vi "UpdateVacPLC.vi"(0 "index of element":i32, 2 "DIMControlMon in (sorted)":refnum<vi>[](array[refnum]), 3 "DIMControlMon out (sorted)":refnum<vi>[](array[refnum]), 4 "Label.Text":string, 5 "Enable?":bool) -> ()   [LabVIEW 2014, in "Panels.lvlib"]
uses:
  Panels.lvlib
  CSCore/CSSystem/CoreDefs/CoreDefs.call_type.ctl
  CSCore/BaseProcess/BaseProcess.descriptor string definition.ctl
  CSCore/CSSystem/CoreDefs/CoreDefs.rawDataType.ctl
  Instance           6 20Saved   UpdateVacPLC .vi
  Instance           7 20Saved   UpdateVacPLC .vi
  Instance           8 20Saved   UpdateVacPLC .vi
  CSCore/CSSystem/CoreLib/CoreLib.short 2 byte array.vi
  Instance           9 20Saved   UpdateVacPLC .vi
  Instance           1 20Saved   UpdateVacPLC .vi
  CSCore/CSSystem/CoreLib/CoreLib.lvlib
  CSCore/BaseProcess/BaseProcess.lvlib
panel:
  in  "call cluster in 2":T1={"Object"="", "Selector"="", "CallType"=enum."synchronous", "Async Object"="", "Async Selector"="", "Data Descriptor"="", "Data"=[], "Error #"=0, "Expire"=0}
  in  "call cluster in":T1={"Object"="", "Selector"="", "CallType"=enum."synchronous", "Async Object"="", "Async Selector"="", "Data Descriptor"="", "Data"=[], "Error #"=0, "Expire"=0}
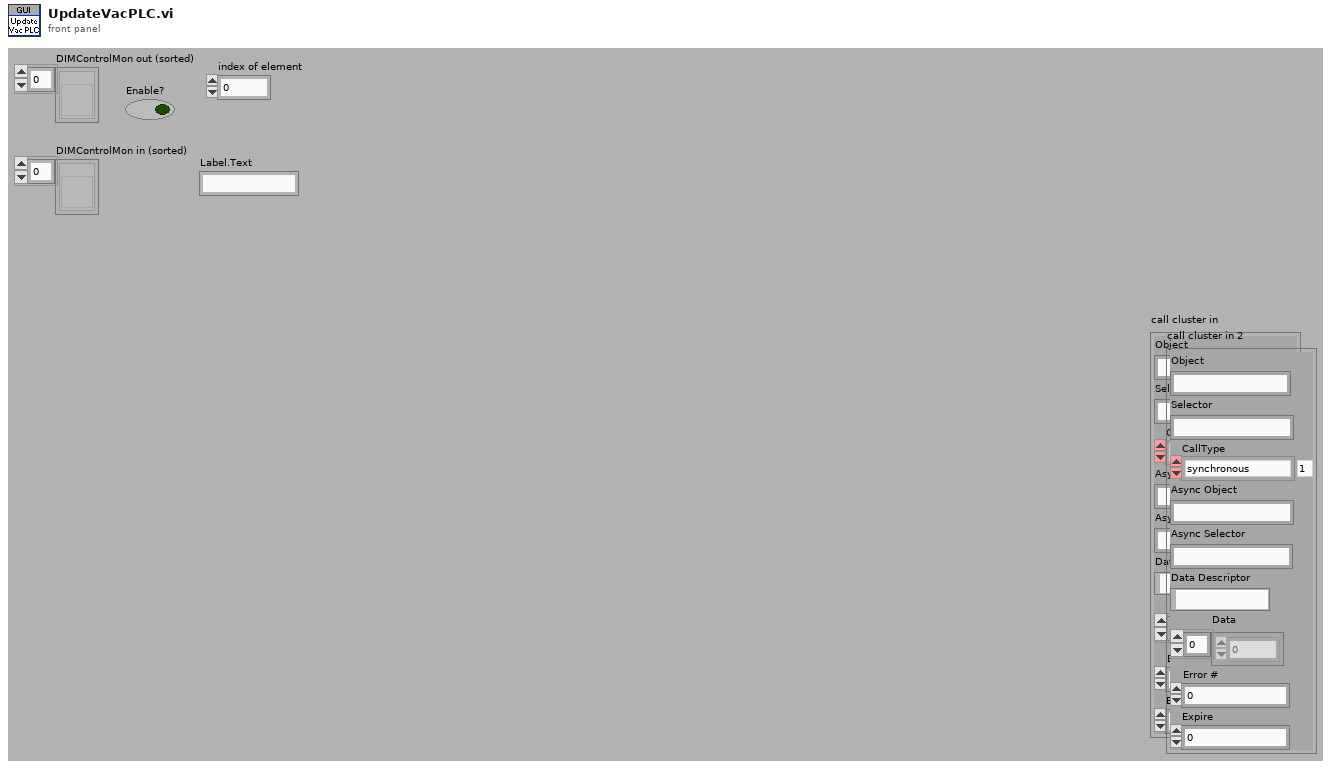
[diagram p1: front panel]
types:
  T1 = typedef "CoreDefs.call_type.ctl" = cluster{"Object":string, "Selector":string, "CallType":enum16{"simple", "synchronous", "asynchronous"}, "Async Object":string, "Async Selector":string, "Data Descriptor":T2, "Data":T3, "Error #":i32, "Expire":u32}
  T2 = typedef "BaseProcess.lvlib/BaseProcess.descriptor string definition.ctl" = string
  T3 = typedef "CoreDefs.rawDataType.ctl" = i8[]
  T4 = cluster{"data":i16, "no link":bool, "quality":i32, "timeStamp":dbl}
  T5 = enum16{"Left Button", "Center Button", "Right Button", "Window Close"}
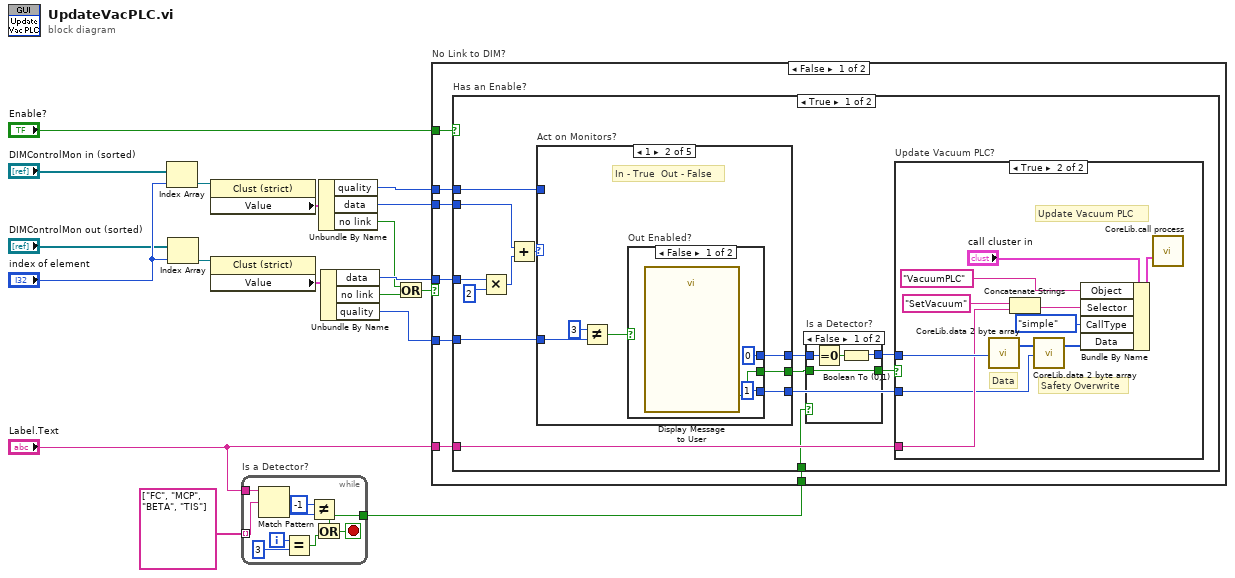
[diagram p0: block diagram]
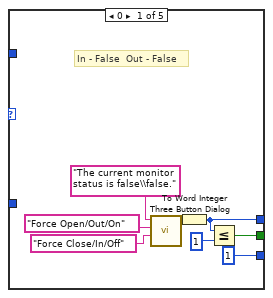
[diagram p4: hidden frame]
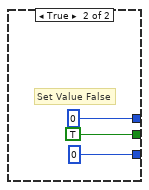
[diagram p5: hidden frame]
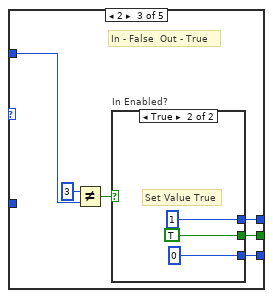
[diagram p6: hidden frame]
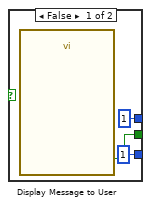
[diagram p7: hidden frame]
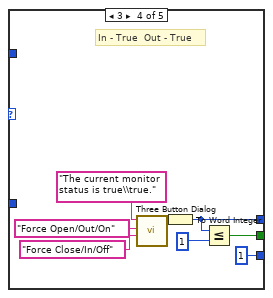
[diagram p8: hidden frame]
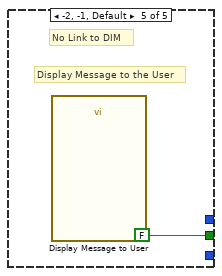
[diagram p9: hidden frame]
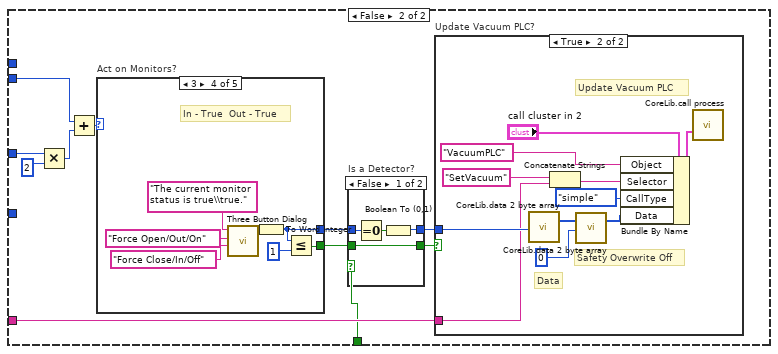
[diagram p10: hidden frame]
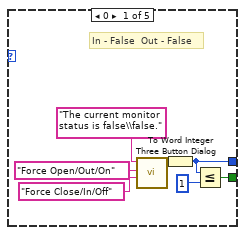
[diagram p13: hidden frame]
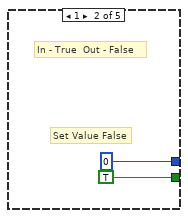
[diagram p14: hidden frame]
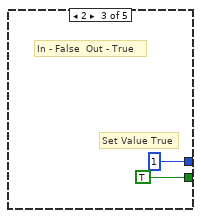
[diagram p15: hidden frame]
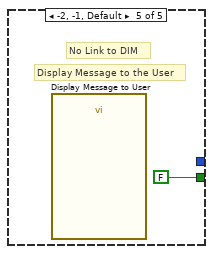
[diagram p16: hidden frame]
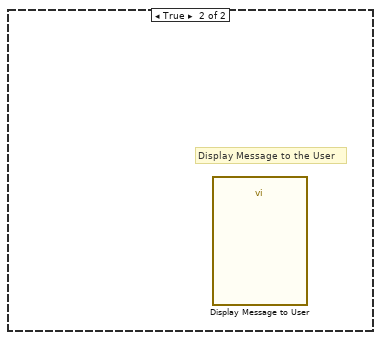
[diagram p17: hidden frame]
diagram:
  n1 = Index Array(array="DIMControlMon in (sorted)", index="index of element") -> (element=w15:refnum<vi>)
  n2 = Index Array(array="DIMControlMon out (sorted)", index="index of element") -> (element=w14:refnum<vi>)
  n3 = property class="Clust (strict)"(reference=w15) -> ("Value"=w13:T4)  [unwired: 1 in, 2 out]
  n4 = property class="Clust (strict)"(reference=w14) -> ("Value"=w12:T4)  [unwired: 1 in, 2 out]
  n5 = while "Is a Detector?" {
    tunnel: string[] ["FC", "MCP", "BETA", "TIS"] -> [w26] mode=indexing
    tunnel: "Label.Text" -> [w27]
    tunnel: [w19] -> w1
    i -> [w25]
    stop <- w21 stop-if-true
    n6 = Match Pattern(string=w27, regular expression=w26) -> (offset past match=w23:i32)  [unwired: 1 in, 3 out]
    n7 = Equal?(x=w25, y=3) -> (x = y?=w20:bool)
    n8 = Not Equal?(x=-1, y=w23) -> (x != y?=w19:bool)
    n9 = Or(x=w19, y=w20) -> (x .or. y?=w21:bool)
  }
  n10 = Unbundle By Name(w13) -> ("quality"=w5:i32, "data"=w10:i16, "no link"=w9:bool)
  n11 = Unbundle By Name(w12) -> ("data"=w11:i16, "no link"=w8:bool, "quality"=w4:i32)
  n12 = Or(x=w9, y=w8) -> (x .or. y?=w7:bool)
  n13 = case "No Link to DIM?" shown="False" w7 {
    tunnel: w11 -> [w34 _]
    tunnel: w10 -> [w33 _]
    tunnel: "Enable?" -> [w32 _]
    tunnel: w5 -> [w31 _]
    tunnel: w4 -> [w30 _]
    tunnel: "Label.Text" -> [w29 _]
    tunnel: w1 -> [w28 _]
    frame False {
      n14 = case "Has an Enable?" shown="True" w32 {
        tunnel: w34 -> [w48 w117]
        tunnel: w33 -> [w45 w114]
        tunnel: w31 -> [w42 _]
        tunnel: w30 -> [w43 _]
        tunnel: w29 -> [w41 w112]
        tunnel: w28 -> [w36 w111]
        frame True {
          n15 = Multiply(x=w48, y=i16 2) -> (x*y=w46:i16)
          n16 = Add(x=w45, y=w46) -> (x+y=w44:i16)
          n17 = case "Act on Monitors?" shown="1" w44 {
            tunnel: [w67 w79 w87 w99 FALSE] -> w39
            tunnel: [w68 w78 w88 w100 _] -> w40
            tunnel: w43 -> [_ w76 _ _ _]
            tunnel: w42 -> [_ _ w89 _ _]
            tunnel: [i16 1 ("i16") w74 w86 i16 1 ("y") _] -> w35
            frame 0 {
              # "In - False  Out - False"
              n18 = call <vilib>:"Three Button Dialog.vi"("Center Button Text (\"No\")"="Force Close/In/Off" ("Left Button Text (\"Yes\")"), "Left Button Text (\"Yes\")"="Force Open/Out/On" ("Left Button Text (\"Yes\")"), "message"="The current monitor status is false\\false.") -> ("Which Button?"=w72:T5)  [unwired: 8 in]
              n19 = To Word Integer(number=w72) -> (16bit integer=w68:i16)
              n20 = Less Or Equal?(x=w68, y=i16 1) -> (x <= y?=w67:bool)
            }
            frame 1 {
              # "In - True  Out - False"
              n21 = Not Equal?(x=3, y=w76) -> (x != y?=w75:bool)
              n22 = case "Out Enabled?" shown="False" w75 {
                tunnel: [w81 TRUE] -> w79
                tunnel: [i16 0 ("y") i16 0 ("y")] -> w78
                tunnel: [i16 1 ("y") i16 0 ("i16")] -> w74
                frame False {
                  n23 = call "Display Message to User"() -> ("OK"=w81:bool)  [unwired: 10 in, 1 out]
                }
                frame True {
                  # "Set Value False"
                }
              }
            }
            frame 2 {
              # "In - False  Out - True"
              n24 = Not Equal?(x=3, y=w89) -> (x != y?=w91:bool)
              n25 = case "In Enabled?" shown="True" w91 {
                tunnel: [w93 TRUE] -> w87
                tunnel: [i16 1 ("y") i16 1 ("y")] -> w88
                tunnel: [i16 1 ("y") i16 0 ("y")] -> w86
                frame False {
                  n26 = call "Display Message to User"() -> ("OK"=w93:bool)  [unwired: 10 in, 1 out]
                }
                frame True {
                  # "Set Value True"
                }
              }
            }
            frame 3 {
              # "In - True  Out - True"
              n27 = call <vilib>:"Three Button Dialog.vi"("Center Button Text (\"No\")"="Force Close/In/Off" ("Left Button Text (\"Yes\")"), "Left Button Text (\"Yes\")"="Force Open/Out/On" ("Left Button Text (\"Yes\")"), "message"="The current monitor status is true\\true.") -> ("Which Button?"=w102:T5)  [unwired: 8 in]
              n28 = To Word Integer(number=w102) -> (16bit integer=w100:i16)
              n29 = Less Or Equal?(x=w100, y=i16 1) -> (x <= y?=w99:bool)
            }
            frame -2, -1, Default {
              # "Display Message to the User"
              # "No Link to DIM"
              n30 = call "Display Message to User"() -> ()  [unwired: 10 in, 2 out]
            }
          }
          n31 = case "Is a Detector?" shown="False" w36 {
            tunnel: w39 -> [w52 w54]
            tunnel: [w52 w54] -> w38
            tunnel: [w51 w53] -> w37
            tunnel: w40 -> [w50 w53]
            frame False {
              n32 = Equal To 0?(x=w50) -> (x = 0?=w49:bool)
              n33 = Boolean To (0,1)(Boolean=w49) -> (0, 1=w51:i16)
            }
            frame True {
            }
          }
          n34 = case "Update Vacuum PLC?" shown="True" w38 {
            tunnel: w37 -> [_ w59]
            tunnel: w41 -> [_ w58]
            tunnel: w35 -> [_ w55]
            frame False {
            }
            frame True {
              # "Data"
              # "Safety Overwrite"
              # "Update Vacuum PLC"
              n35 = call-poly "CoreLib.data 2 byte array.vi"("i16"=w59) -> ("byteArray out"=w57:T3)  [unwired: 18 in]
              n36 = Concatenate Strings("SetVacuum" ("string"), w58) -> (w61:string)
              n37 = call-poly "CoreLib.data 2 byte array.vi"("byteArray"=w57, "i16"=w55) -> ("byteArray out"=w56:T3)  [unwired: 17 in]
              n38 = Bundle By Name(cluster="call cluster in", "Object"="VacuumPLC", "Selector"=w61, "CallType"=enum16{"simple", "synchronous", "asynchronous"}."simple", "Data"=w56) -> (w64:T1)
              n39 = call "CoreLib.call process.vi"("call cluster in"=w64) -> ()  [unwired: 13 in, 2 out]
            }
          }
        }
        frame False {
          n40 = Multiply(x=w117, y=i16 2) -> (x*y=w115:i16)
          n41 = Add(x=w114, y=w115) -> (x+y=w113:i16)
          n42 = case "Act on Monitors?" shown="3" w113 {
            tunnel: [w138 TRUE TRUE w147 FALSE] -> w110
            tunnel: [w136 i16 0 ("y") i16 1 ("y") w146 _] -> w108
            frame 0 {
              # "In - False  Out - False"
              n43 = call <vilib>:"Three Button Dialog.vi"("Center Button Text (\"No\")"="Force Close/In/Off" ("Left Button Text (\"Yes\")"), "Left Button Text (\"Yes\")"="Force Open/Out/On" ("Left Button Text (\"Yes\")"), "message"="The current monitor status is false\\false.") -> ("Which Button?"=w137:T5)  [unwired: 8 in]
              n44 = To Word Integer(number=w137) -> (16bit integer=w136:i16)
              n45 = Less Or Equal?(x=w136, y=i16 1) -> (x <= y?=w138:bool)
            }
            frame 1 {
              # "Set Value False"
              # "In - True  Out - False"
            }
            frame 2 {
              # "Set Value True"
              # "In - False  Out - True"
            }
            frame 3 {
              # "In - True  Out - True"
              n46 = call <vilib>:"Three Button Dialog.vi"("Center Button Text (\"No\")"="Force Close/In/Off" ("Left Button Text (\"Yes\")"), "Left Button Text (\"Yes\")"="Force Open/Out/On" ("Left Button Text (\"Yes\")"), "message"="The current monitor status is true\\true.") -> ("Which Button?"=w151:T5)  [unwired: 8 in]
              n47 = To Word Integer(number=w151) -> (16bit integer=w146:i16)
              n48 = Less Or Equal?(x=w146, y=i16 1) -> (x <= y?=w147:bool)
            }
            frame -2, -1, Default {
              # "Display Message to the User"
              # "No Link to DIM"
              n49 = call "Display Message to User"() -> ()  [unwired: 10 in, 2 out]
            }
          }
          n50 = case "Is a Detector?" shown="False" w111 {
            tunnel: w110 -> [w121 w123]
            tunnel: [w121 w123] -> w109
            tunnel: [w120 w122] -> w107
            tunnel: w108 -> [w119 w122]
            frame False {
              n51 = Equal To 0?(x=w119) -> (x = 0?=w118:bool)
              n52 = Boolean To (0,1)(Boolean=w118) -> (0, 1=w120:i16)
            }
            frame True {
            }
          }
          n53 = case "Update Vacuum PLC?" shown="True" w109 {
            tunnel: w107 -> [_ w128]
            tunnel: w112 -> [_ w127]
            frame False {
            }
            frame True {
              # "Data"
              # "Safety Overwrite Off"
              # "Update Vacuum PLC"
              n54 = call-poly "CoreLib.data 2 byte array.vi"("i16"=w128) -> ("byteArray out"=w125:T3)  [unwired: 18 in]
              n55 = Concatenate Strings("SetVacuum" ("string"), w127) -> (w130:string)
              n56 = call-poly "CoreLib.data 2 byte array.vi"("byteArray"=w125, "i16"=i16 0) -> ("byteArray out"=w126:T3)  [unwired: 17 in]
              n57 = Bundle By Name(cluster="call cluster in 2", "Object"="VacuumPLC", "Selector"=w130, "CallType"=enum16{"simple", "synchronous", "asynchronous"}."simple", "Data"=w126) -> (w133:T1)
              n58 = call "CoreLib.call process.vi"("call cluster in"=w133) -> ()  [unwired: 13 in, 2 out]
            }
          }
        }
      }
    }
    frame True {
      # "Display Message to the User"
      n59 = call "Display Message to User"() -> ()  [unwired: 10 in, 2 out]
    }
  }
